vi "获取最近两组水样测试数据.vi"(8 "error in (no error)":errorcluster, 10 "运行模式":enum16{"维护模式", "常规模式", "应急模式", "质控模式"}(ring), 11 "table":string) -> (0 "error out":errorcluster, 3 "存储变量":T1={"时间标识"=timestamp(0 s since 1904-01-01), "参数"="", "数据类型"="N", "集成干预测试浓度值"=0.0, "集成干预前测试时间"=timestamp(0 s since 1904-01-01), "集成干预前测试浓度值"=0.0})   [LabVIEW 2016, in "PLC.lvlib"]
uses:
  PLC.lvlib
  <vilib>/Utility/sysdir.llb/System Directory Type.ctl
  <vilib>/addons/database/Connection.llb/DB Tools Open Connec (String).vi
  <vilib>/addons/database/Connection.llb/Conn Execute.vi
  <vilib>/addons/database/Recordset.llb/Rec Fetch Recordset Data (R).vi
  <vilib>/addons/database/Recordset.llb/Rec Destroy - Connection.vi
  <vilib>/addons/database/_DB Variant To Data/Database Variant To Data.xnode
  <vilib>/addons/database/NI_Database_API.lvlib
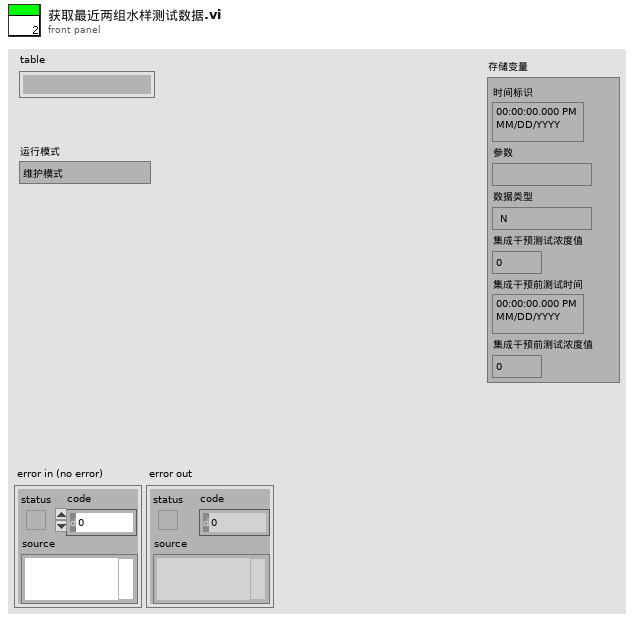
[diagram p1: front panel]
types:
  T1 = cluster{"时间标识":timestamp, "参数":string, "数据类型":string, "集成干预测试浓度值":dbl, "集成干预前测试时间":timestamp, "集成干预前测试浓度值":dbl}
  T2 = typedef "System Directory Type.ctl" = i32
  T3 = typedef "NI_Database_API.lvlib/Conn ObjectReference.ctl" = refnum<k1>
  T4 = typedef "NI_Database_API.lvlib/Rec ObjectReference.ctl" = refnum<k1>
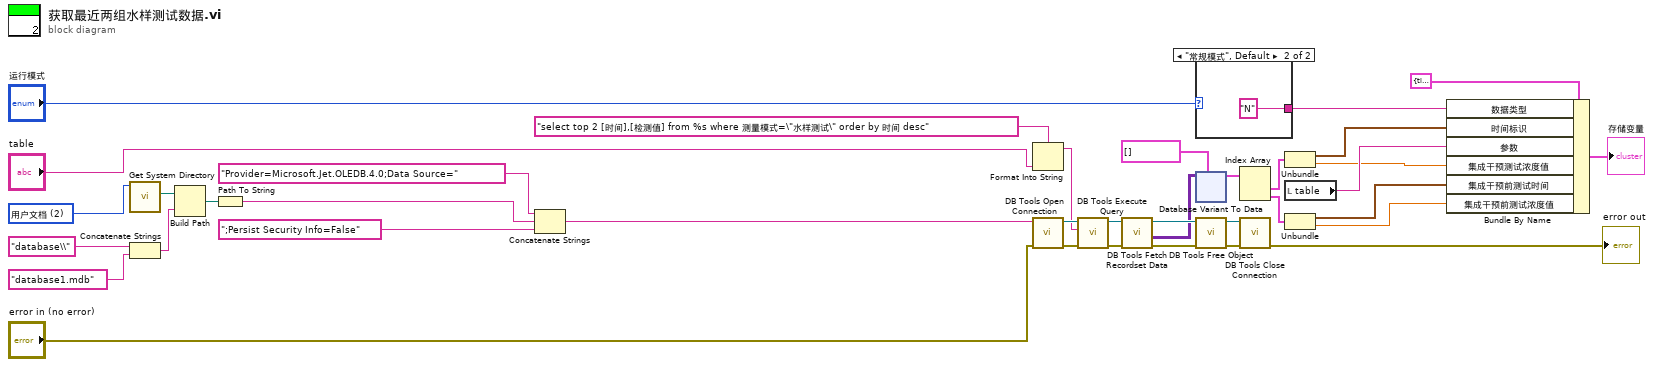
[diagram p0: block diagram]
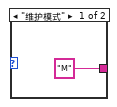
[diagram p2: hidden frame]
diagram:
  w35 = T2 2 items=["用户目录"=0, "用户桌面"=1, "用户文档"=2, "用户应用程序数据"=3, "用户设置"=4, "用户临时目录"=5, "公共文档"=6, "公共应用程序数据"=7, "公共设置"=8, "公共缓存"=13, "系统核心库"=9, "系统安装库"=10, "应用程序文件"=11, "启动盘根目录"=12] ("system directory type")
  n1 = call <vilib>:"Get System Directory.vi"("system directory type"=w35) -> ("system directory"=w33:path)  [unwired: 10 in]
  n2 = Concatenate Strings("database\\" ("condition"), "database1.mdb" ("condition")) -> (w27:string)
  n3 = Build Path(base path=w33, name or relative path=w27) -> (appended path=w32:path)
  n4 = Path To String(path=w32) -> (string=w31:string)
  n5 = Concatenate Strings("Provider=Microsoft.Jet.OLEDB.4.0;Data Source=" ("condition"), w31, ";Persist Security Info=False" ("condition")) -> (w29:string)
  n6 = Format Into String(format string="select top 2 [时间],[检测值] from %s where 测量模式=\"水样测试\" order by 时间 desc" ("格式字符串"), "table") -> (resulting string=w16:string)  [unwired: 2 in, 1 out]
  n7 = call-poly <vilib>:"DB Tools Open Connection.vi"("error in (no error)"="error in (no error)", "connection information"=w29) -> ("error out"=w22:errorcluster, "connection reference"=w23:T3)  [unwired: 6 in]
  n8 = call-poly <vilib>:"DB Tools Execute Query.vi"("error in (no error)"=w22, "SQL query"=w16, "connection reference"=w23) -> ("error out"=w21:errorcluster, "recordset reference"=w26:T4)  [unwired: 5 in]
  n9 = call-poly <vilib>:"DB Tools Fetch Recordset Data.vi"("error in (no error)"=w21, "recordset reference"=w26) -> ("error out"=w24:errorcluster, "recordset data"=w14:variant[][], "recordset reference out"=w25:T4)  [unwired: 3 in]
  n10 = case shown="\"常规模式\", Default" "运行模式" {
    tunnel: ["M" "N"] -> w1
    frame "维护模式" {
    }
    frame "常规模式", Default {
    }
  }
  n11 = xnode "Database Variant To Data"("database variant"=w14, "type"=cluster{"时间":timestamp, "检测值 ":dbl}[] []) -> ("data"=w11:cluster{timestamp, dbl}[])  [unwired: 1 in, 1 out]
  n12 = call-poly <vilib>:"DB Tools Free Object.vi"("error in (no error)"=w24, "recordset reference"=w25) -> ("error out"=w19:errorcluster, "connection reference"=w20:T3)  [unwired: 8 in]
  n13 = Index Array(array=w11) -> (element #1=w10:cluster{timestamp, dbl}, element #2=w7:cluster{timestamp, dbl})  [unwired: 2 in]
  n14 = call <vilib>:"DB Tools Close Connection.vi"("error in (no error)"=w19, "connection reference"=w20) -> ("error out"=→"error out":errorcluster)  [unwired: 5 in]
  n15 = Unbundle(w10) -> (w9:timestamp, w8:dbl)
  n16 = local read "table"() -> (w12:string)
  n17 = Unbundle(w7) -> (w6:timestamp, w5:dbl)
  n18 = Bundle By Name(cluster=T1 {"时间标识"=timestamp(0 s since 1904-01-01), "参数"="", "数据类型"="N", "集成干预测试浓度值"=0.0, "集成干预前测试时间"=timestamp(0 s since 1904-01-01), "集成干预前测试浓度值"=0.0} ("存储变量"), "数据类型"=w1, "时间标识"=w9, "参数"=w12, "集成干预测试浓度值"=w8, "集成干预前测试时间"=w6, "集成干预前测试浓度值"=w5) -> (→"存储变量":T1)
